vi "capacitor.vi"(1 "Invert Y":bool, 2 "Invert X":bool, 4 "L2":dbl=2.0, 5 "L3":dbl=1.0, 6 "Swap-XY":bool, 7 "L1":dbl=1.0, 8 "Device in Y":refnum<k24>, 9 "GetPOS Y":refnum<vi>, 10 "GetPOS X":refnum<vi>, 11 "Device in X":refnum<k24>) -> (0 "Device out Y":refnum<k24>, 3 "Device out X":refnum<k24>)   [LabVIEW 2014]
doc: "André Romero - 2019\nandretec@ifsc.usp.br"
uses:
  C:/users-lab/Andre/GITs/andretec/Thorlabs-Vector-Move/kinesisTec/Kinesis/Thorlabs.MotionControl.TCube.DCServoCLI.dll
  Kinesis/Thorlabs.MotionControl.TCube.DCServoCLI.dll
  motorsGlobalVar.vi
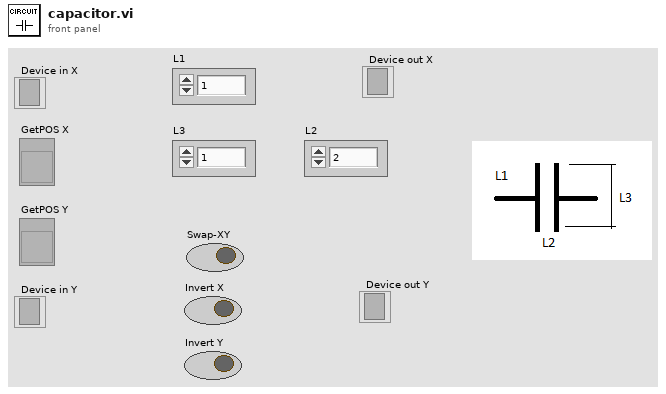
[diagram p1: front panel]
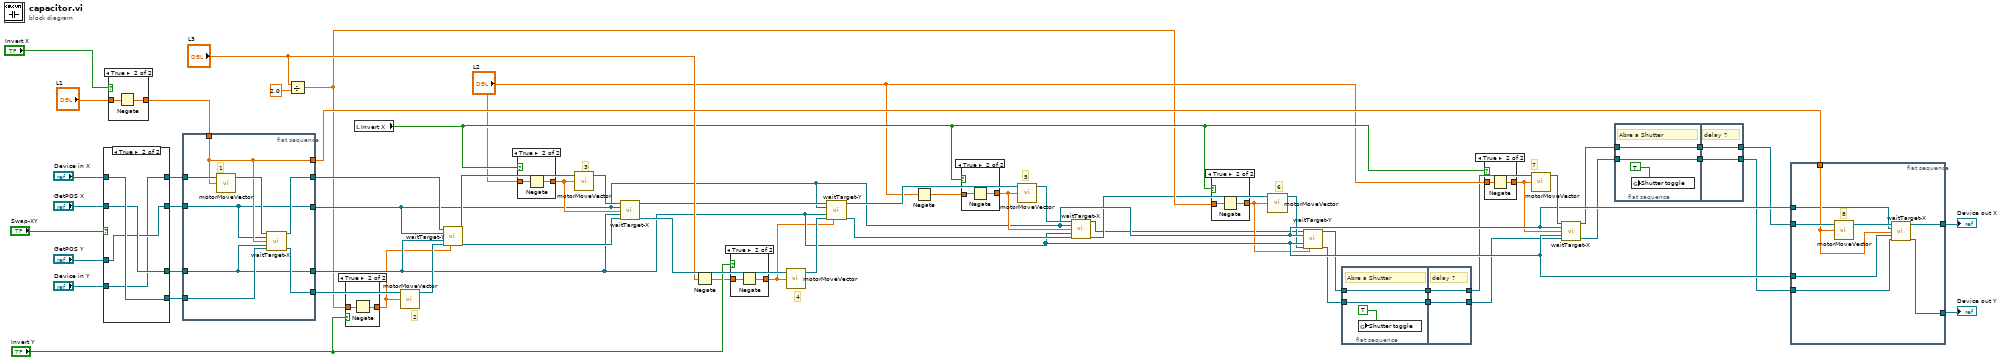
[diagram p0: block diagram]
diagram:
  # "7"
  # "6"
  # "5"
  # "4"
  # "3"
  # "2"
  n1 = case shown="True" "Swap-XY" {
    tunnel: "Device in X" -> [w61 w67]
    tunnel: [w61 w64] -> w53
    tunnel: "GetPOS Y" -> [w63 w65]
    tunnel: [w63 w66] -> w51
    tunnel: "Device in Y" -> [w62 w64]
    tunnel: [w62 w67] -> w49
    tunnel: "GetPOS X" -> [w60 w66]
    tunnel: [w60 w65] -> w47
    frame False {
    }
    frame True {
    }
  }
  n2 = case shown="True" "Invert X" {
    tunnel: "L1" -> [w68 w70]
    tunnel: [w68 w69] -> w42
    frame False {
    }
    frame True {
      n3 = Negate(x=w70) -> (-x=w69:dbl)
    }
  }
  n4 = flat-sequence {
    tunnel: w53 -> [w78]
    tunnel: [w75] -> w40
    tunnel: w49 -> [w76]
    tunnel: [w74] -> w58
    tunnel: [w72] -> w24
    tunnel: [w71] -> w22
    tunnel: [w73] -> w59
    tunnel: w42 -> [w73]
    tunnel: w47 -> [w72]
    tunnel: w51 -> [w71]
    frame #0 {
      # "1"
      n5 = call "motorMoveVector.vi"("Distance"=w73, "Device in"=w78) -> ("Device out"=w77:refnum<k24>)  [unwired: 3 in]
      n6 = call "waitTarget-X.vi"("Device in X"=w77, "GetPOS X"=w72, "Position X"=w73, "GetPOS Y"=w71, "Device in Y"=w76) -> ("Device out X"=w75:refnum<k24>, "Device out Y"=w74:refnum<k24>)  [unwired: 7 in, 2 out]
    }
  }
  n7 = Divide(x="L3", y=2.0) -> (x/y=w18:dbl)
  n8 = case shown="True" "Invert Y" {
    tunnel: w18 -> [w79 w81]
    tunnel: [w79 w80] -> w21
    frame False {
    }
    frame True {
      n9 = Negate(x=w81) -> (-x=w80:dbl)
    }
  }
  n10 = local read "Invert X"() -> (w25:bool)
  n11 = call "motorMoveVector.vi"("Distance"=w21, "Device in"=w58) -> ("Device out"=w57:refnum<k24>)  [unwired: 3 in]
  n12 = call "waitTarget-Y.vi"("Device in X"=w40, "GetPOS X"=w24, "GetPOS Y"=w22, "Device in Y"=w57, "Position Y"=w21) -> ("Device out X"=w39:refnum<k24>, "Device out Y"=w37:refnum<k24>)  [unwired: 7 in, 2 out]
  n13 = case shown="True" w25 {
    tunnel: [w82 w83] -> w36
    tunnel: "L2" -> [w82 w84]
    frame False {
    }
    frame True {
      n14 = Negate(x=w84) -> (-x=w83:dbl)
    }
  }
  n15 = call "motorMoveVector.vi"("Distance"=w36, "Device in"=w39) -> ("Device out"=w38:refnum<k24>)  [unwired: 3 in]
  n16 = call "waitTarget-X.vi"("Device in X"=w38, "GetPOS X"=w24, "Position X"=w36, "GetPOS Y"=w22, "Device in Y"=w37) -> ("Device out X"=w32:refnum<k24>, "Device out Y"=w35:refnum<k24>)  [unwired: 7 in, 2 out]
  n17 = Negate(x="L3") -> (-x=w19:dbl)
  n18 = case shown="True" "Invert Y" {
    tunnel: [w85 w86] -> w20
    tunnel: w19 -> [w85 w87]
    frame False {
    }
    frame True {
      n19 = Negate(x=w87) -> (-x=w86:dbl)
    }
  }
  n20 = call "motorMoveVector.vi"("Distance"=w20, "Device in"=w35) -> ("Device out"=w33:refnum<k24>)  [unwired: 3 in]
  n21 = call "waitTarget-Y.vi"("Device in X"=w32, "GetPOS X"=w24, "GetPOS Y"=w22, "Device in Y"=w33, "Position Y"=w20) -> ("Device out X"=w30:refnum<k24>, "Device out Y"=w26:refnum<k24>)  [unwired: 7 in, 2 out]
  n22 = Negate(x="L2") -> (-x=w29:dbl)
  n23 = case shown="True" w25 {
    tunnel: [w88 w89] -> w27
    tunnel: w29 -> [w88 w90]
    frame False {
    }
    frame True {
      n24 = Negate(x=w90) -> (-x=w89:dbl)
    }
  }
  n25 = call "motorMoveVector.vi"("Distance"=w27, "Device in"=w30) -> ("Device out"=w28:refnum<k24>)  [unwired: 3 in]
  n26 = call "waitTarget-X.vi"("Device in X"=w28, "GetPOS X"=w24, "Position X"=w27, "GetPOS Y"=w22, "Device in Y"=w26) -> ("Device out X"=w13:refnum<k24>, "Device out Y"=w15:refnum<k24>)  [unwired: 7 in, 2 out]
  n27 = case shown="True" w25 {
    tunnel: [w91 w92] -> w17
    tunnel: w18 -> [w91 w93]
    frame False {
    }
    frame True {
      n28 = Negate(x=w93) -> (-x=w92:dbl)
    }
  }
  n29 = call "motorMoveVector.vi"("Distance"=w17, "Device in"=w15) -> ("Device out"=w14:refnum<k24>)  [unwired: 3 in]
  n30 = call "waitTarget-Y.vi"("Device in X"=w13, "GetPOS X"=w24, "GetPOS Y"=w22, "Device in Y"=w14, "Position Y"=w17) -> ("Device out X"=w10:refnum<k24>, "Device out Y"=w8:refnum<k24>)  [unwired: 7 in, 2 out]
  n31 = flat-sequence {
    tunnel: w10 -> [w96]
    tunnel: w8 -> [w95]
    tunnel: [w96] -> w12
    tunnel: [w95] -> w11
    tunnel: [w97] -> w7
    tunnel: [w98] -> w9
    tunnel: w12 -> [w98]
    tunnel: w11 -> [w97]
    frame #0 {
      # "Abre a Shutter"
      n32 = global write "motorsGlobalVar.vi" "Shutter toggle"(TRUE ("Shutter toggle")) -> ()
    }
    frame #1 {
      # "delay ?"
    }
  }
  n33 = case shown="True" w25 {
    tunnel: [w99 w100] -> w16
    tunnel: "L2" -> [w99 w101]
    frame False {
    }
    frame True {
      n34 = Negate(x=w101) -> (-x=w100:dbl)
    }
  }
  n35 = call "motorMoveVector.vi"("Distance"=w16, "Device in"=w9) -> ("Device out"=w55:refnum<k24>)  [unwired: 3 in]
  n36 = call "waitTarget-X.vi"("Device in X"=w55, "GetPOS X"=w24, "Position X"=w16, "GetPOS Y"=w22, "Device in Y"=w7) -> ("Device out X"=w4:refnum<k24>, "Device out Y"=w2:refnum<k24>)  [unwired: 7 in, 2 out]
  n37 = flat-sequence {
    tunnel: w4 -> [w104]
    tunnel: w2 -> [w103]
    tunnel: [w104] -> w6
    tunnel: [w103] -> w5
    tunnel: [w105] -> w1
    tunnel: [w106] -> w3
    tunnel: w6 -> [w106]
    tunnel: w5 -> [w105]
    frame #0 {
      # "Abre a Shutter"
      n38 = global write "motorsGlobalVar.vi" "Shutter toggle"(TRUE ("Shutter toggle")) -> ()
    }
    frame #1 {
      # "delay ?"
    }
  }
  n39 = flat-sequence {
    tunnel: w3 -> [w114]
    tunnel: w1 -> [w109]
    tunnel: [w108] -> w44
    tunnel: w22 -> [w112]
    tunnel: w59 -> [w111]
    tunnel: [w110] -> w45
    tunnel: w24 -> [w107]
    frame #0 {
      # "8"
      n40 = call "motorMoveVector.vi"("Distance"=w111, "Device in"=w114) -> ("Device out"=w113:refnum<k24>)  [unwired: 3 in]
      n41 = call "waitTarget-X.vi"("Device in X"=w113, "GetPOS X"=w107, "Position X"=w111, "GetPOS Y"=w112, "Device in Y"=w109) -> ("Device out X"=w110:refnum<k24>, "Device out Y"=w108:refnum<k24>)  [unwired: 7 in, 2 out]
    }
  }
  "Device out X" <- w45
  "Device out Y" <- w44
